vi "svfa_Scaled Time Domain Window (1 Ch).vi"(0 "Signal in [X]":waveform(dbl)={"t0"=timestamp(0 s since 1904-01-01), "dt"=1.953125e-05, "Y"=[]}, 5 "window":T1 items=["None"=0, "Hanning"=1, "Hamming"=2, "Blackman-Harris"=3, "Exact Blackman"=4, "Blackman"=5, "Flat Top"=6, "4 Term B-Harris "=7, "7 Term B-Harris"=8, "Low Sidelobe"=9, "Force"=64, "Exponential"=65, "Blackman Nuttall"=11, "Triangle"=30, "Bartlett-Hanning"=31, "Bohman"=32, "Parzen"=33, "Welch"=34, "Kaiser"=60, "Dolph-Chebyshev"=61, "Gaussian"=62], 7 "window parameter":dbl=nan format="%0.2f", 11 "error in":errorcluster) -> (4 "Windowed Waveform":waveform(dbl), 6 "dup window":T1 items=["None"=0, "Hanning"=1, "Hamming"=2, "Blackman-Harris"=3, "Exact Blackman"=4, "Blackman"=5, "Flat Top"=6, "4 Term B-Harris "=7, "7 Term B-Harris"=8, "Low Sidelobe"=9, "Force"=64, "Exponential"=65, "Blackman Nuttall"=11, "Triangle"=30, "Bartlett-Hanning"=31, "Bohman"=32, "Parzen"=33, "Welch"=34, "Kaiser"=60, "Dolph-Chebyshev"=61, "Gaussian"=62], 8 "window length":i32, 10 "FFT length":i32, 13 "window constants":cluster{"ENBW":dbl, "CG":dbl} {"CG" format="%.2f"; "ENBW" format="%.2f"}, 15 "error out":errorcluster)   [LabVIEW 2017]
doc: "Applies the selected window to the time-domain signal. The VI scales the result so that when the power or amplitude spectrum of the windowed waveform is computed, all windows provide the same level within the accuracy constraints of the window."
uses:
  <vilib>/addons/_NISVFA/_Shared subVIs/Controls/svc_Window.ctl
  <vilib>/Analysis/4window.llb/Force Window.vi
  <vilib>/Analysis/4window.llb/Force Window (DBL).vi
  <vilib>/Analysis/4window.llb/Exponential Window.vi
  <vilib>/Analysis/4window.llb/Exponential Window (DBL).vi
  <vilib>/Utility/error.llb/Error Cluster From Error Code.vi
  <vilib>/Analysis/0measdsp.llb/Scaled Time Domain Window.vi
  <vilib>/Analysis/0measdsp.llb/Scaled Time Domain Window (DBL).vi
  <vilib>/addons/_NISVFA/_Spectrum Processing/subVIs/svfa_Spectrum Info Window to windowTd Type Def.vi
panel:
  # "Scaled Time Domain Window"
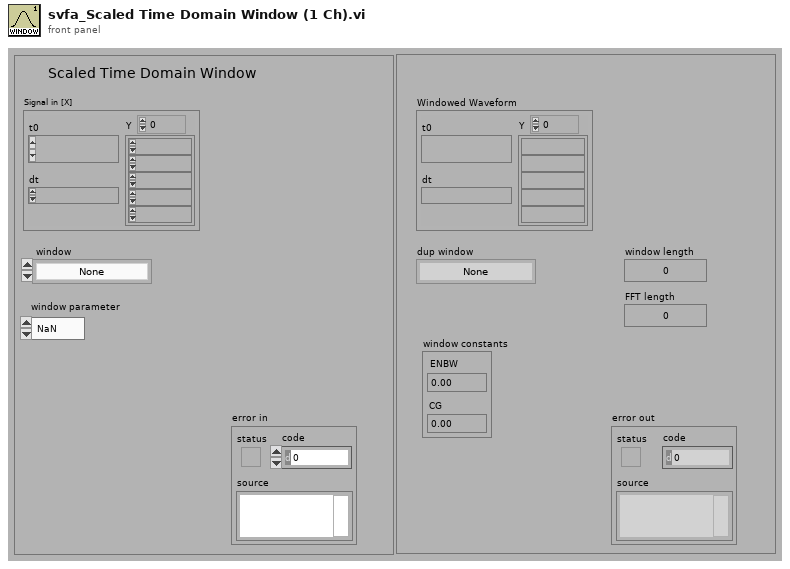
[diagram p1: front panel]
types:
  T1 = typedef "svc_Window.ctl" = u32
  T2 = typedef "NI_AALPro.lvlib/windowTd.ctl" = u32
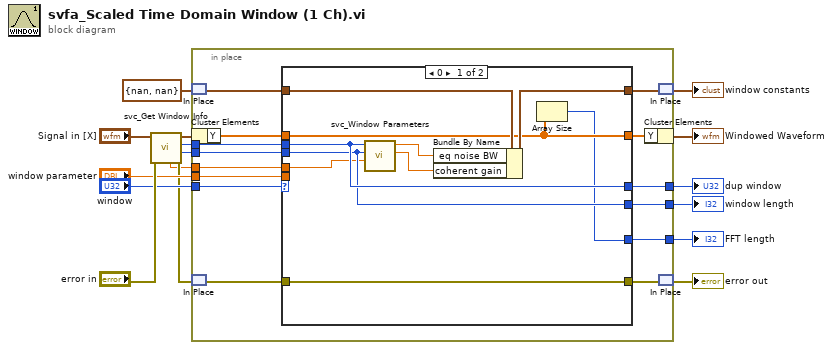
[diagram p0: block diagram]
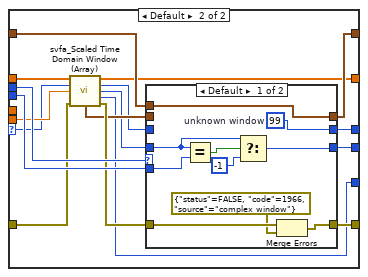
[diagram p2: hidden frame]
diagram:
  n1 = call <vilib>:"svc_Get Window Info.vi"("error in (no error)"="error in", "scaled signal [EU]"="Signal in [X]") -> ("error out"=w5:errorcluster, "window size"=w9:i32, "window"=w10:T2, "dup scaled signal [EU]"=w7:waveform(dbl), "window parameter"=w1:dbl)  [unwired: 5 in]
  n2 = in-place {
    in-place-border: "window" -> [w30]
    in-place-border: [w29] -> w13
    in-place-border: [w28] -> w12
    in-place-border: "window parameter" -> [w27]
    in-place-border: w10 -> [w26]
    in-place-border: w9 -> [w25]
    in-place-border: [w24] -> w8
    in-place-border: w1 -> [w17]
    n3 = in-place-match #1(cluster{"eq noise BW":dbl, "coherent gain":dbl} {"eq noise BW"=nan, "coherent gain"=nan} ("window properties")) -> (w19:cluster{"eq noise BW":dbl, "coherent gain":dbl})
    n4 = in-place-cluster #2(w7) -> ("Y"=w20:dbl[])
    n5 = in-place-match #3(w5) -> (w22:errorcluster)
    n6 = case shown="0" w30 {
      selector: w30 -> [_ w43]
      tunnel: [w34 w54] -> w18
      tunnel: [w32 w49] -> w23
      tunnel: [w37 w55] -> w28
      tunnel: w26 -> [w38 w57]
      tunnel: w25 -> [w37 w53]
      tunnel: [w38 w56] -> w29
      tunnel: w27 -> [_ w48]
      tunnel: [w36 w52] -> w21
      tunnel: w22 -> [w36 w47]
      tunnel: w19 -> [w35 w51]
      tunnel: [w31 w41] -> w24
      tunnel: w20 -> [w32 w50]
      tunnel: w17 -> [w33 _]
      frame 0 {
        n7 = call <vilib>:"svc_Window Parameters.vi"("standard deviation"=w33, "window size"=w37, "window"=w38) -> ("Coherent Gain"=w39:dbl, "ENBW"=w40:dbl)  [unwired: 5 in, 2 out]
        n8 = Bundle By Name(cluster=w35, "eq noise BW"=w40, "coherent gain"=w39) -> (w34:cluster{"eq noise BW":dbl, "coherent gain":dbl})
        n9 = Array Size(array=w32) -> (size(s)=w31:i32)
      }
      frame Default {
        n10 = call <vilib>:"svfa_Scaled Time Domain Window (Array).vi"("input signal"=w50, "window"=w43, "window parameter"=w48, "error in"=w47) -> ("windowed signal"=w49:dbl[], "dup window"=w42:T1, "window length"=w44:i32, "FFT length"=w41:i32, "window constants"=w45:cluster{"ENBW":dbl, "CG":dbl}, "error out"=w46:errorcluster)  [unwired: 6 in]
        n11 = case shown="Default" w57 {
          tunnel: w44 -> [w66 w70]
          tunnel: w42 -> [_ w71]
          tunnel: [w59 w71] -> w56
          tunnel: [w65 w70] -> w55
          tunnel: w45 -> [_ w69]
          tunnel: [w60 w69] -> w54
          tunnel: w53 -> [w67 _]
          tunnel: [w61 w68] -> w52
          tunnel: w46 -> [w62 w68]
          tunnel: w51 -> [w60 _]
          frame Default {
            w59 = u32 99  # unknown window
            n12 = Equal?(x=w66, y=w67) -> (x = y?=w64:bool)
            n13 = Select(t=w66, s=w64, f=-1) -> (s? t:f=w65:i32)
            n14 = Merge Errors(w62, errorcluster {"status"=FALSE, "code"=1966, "source"="complex window"} ("error in 2 (no error)")) -> (w61:errorcluster)
          }
          frame 0 {
          }
        }
      }
    }
    n15 = in-place-cluster #2("Y"=w23) -> (→"Windowed Waveform":waveform(dbl))
    n16 = in-place-match #1(w18) -> (→"window constants":cluster{"eq noise BW":dbl, "coherent gain":dbl})
    n17 = in-place-match #3(w21) -> (→"error out":errorcluster)
  }
  "window length" <- w12
  "dup window" <- w13
  "FFT length" <- w8
